vi "Start and Forget FP.vi"(8 "error in":errorcluster, 11 "Pcal GUI in":refnum<class "Pcal GUI.lvclass">) -> (0 "error out":errorcluster, 1 "Stop":refnum<user-event>, 2 "UI Ref":refnum<vi>, 3 "Pcal GUI out":refnum<class "Pcal GUI.lvclass">)   [LabVIEW 2013, in "Pcal GUI.lvclass"]
uses:
  Pcal GUI.lvclass
  Reusable/GUI/GUI.lvclass
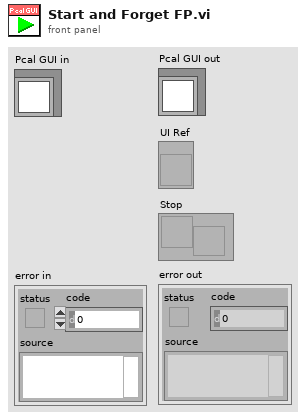
[diagram p1: front panel]
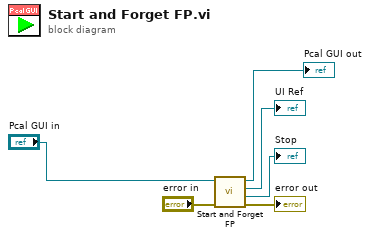
[diagram p0: block diagram]
diagram:
  n1 = call-parent "Start and Forget FP.vi"("error in"="error in", "GUI in"="Pcal GUI in") -> ("error out"=→"error out":errorcluster, "Stop"=→"Stop":refnum<user-event>, "UI Ref"=→"UI Ref":refnum<vi>, "GUI out"=→"Pcal GUI out":refnum<class "Pcal GUI.lvclass">)  [unwired: 6 in]
